vi "Find Connected Resources.vi"(8 "error in (no error)":errorcluster, 9 "Return Aliases":bool=TRUE, 10 "Search Expression":string="?*", 11 "AbstractResourceEnumerator in":refnum<class "AbstractResourceEnumerator.lvclass">) -> (0 "error out":errorcluster, 2 "Found Resources":string[](array[string]), 3 "AbstractResourceEnumerator out":refnum<class "AbstractResourceEnumerator.lvclass">)   [LabVIEW 2023, in "HAF.lvlib" / "AbstractResourceEnumerator.lvclass"]
doc: "Builds a collection of names of resources currently connected to the System. If Return Aliases is True, then only resources with an Alias are returned - any connected resource without an alias is ignored. If Return Aliases is False then the collection will be for all connected resources."
uses:
  AbstractResourceEnumerator.lvclass
  AbstractResourceEnumerator.lvclass/AbstractResourceEnumerator.ctl
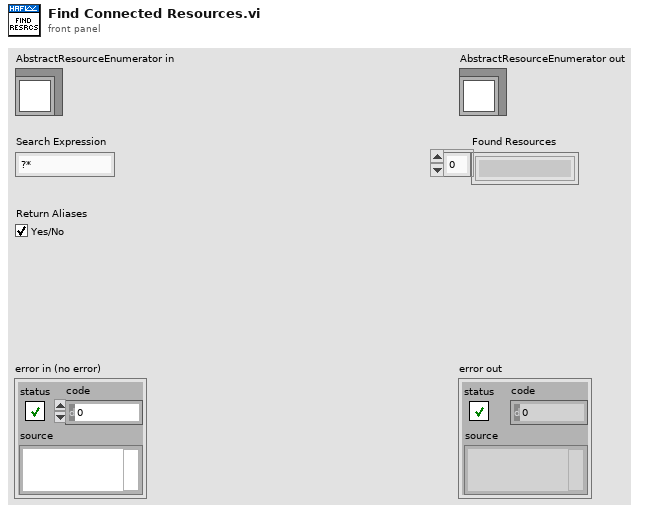
[diagram p1: front panel]
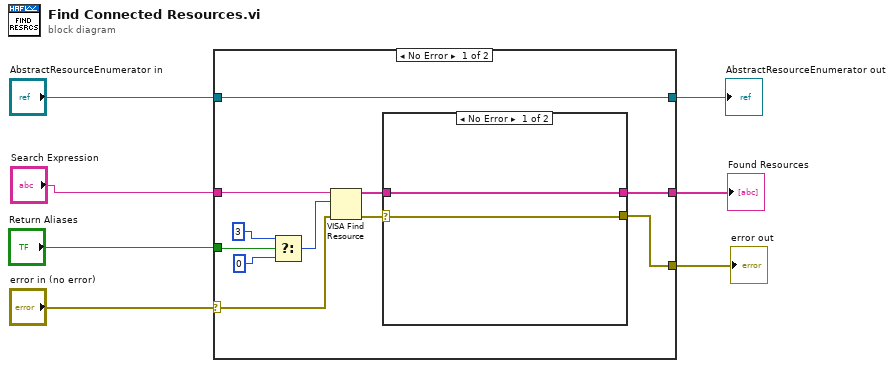
[diagram p0: block diagram]
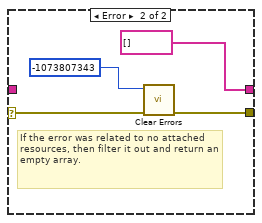
[diagram p2: hidden frame]
diagram:
  n1 = case shown="No Error" "error in (no error)" {
    selector: "error in (no error)" -> [w13 w25]
    tunnel: [w11 w26] -> w3
    tunnel: "AbstractResourceEnumerator in" -> [w11 w26]
    tunnel: "Return Aliases" -> [w18 _]
    tunnel: "Search Expression" -> [w15 _]
    tunnel: [w10 _] -> w2
    tunnel: [w9 w25] -> w1
    frame No Error {
      n2 = Select(t=u32 3, s=w18, f=u32 0) -> (s? t:f=w14:u32)
      n3 = VISA Find Resource(8:w13, 10:w14, 11:w15) -> (0:w8:errorcluster, 3:w12:string[])  [unwired: 1 out]
      n4 = case shown="No Error" w8 {
        selector: w8 -> [w19 w23]
        tunnel: [w19 w22] -> w9
        tunnel: [w20 string[] []] -> w10
        tunnel: w12 -> [w20 _]
        frame No Error {
        }
        frame Error {
          # "If the error was related to no attached resources, then filter it out and return an empty array."
          n5 = call <vilib>:"Clear Errors.vi"("error in (no error)"=w23, "specific error code to clear (0: all)"=-1073807343) -> ("error out"=w22:errorcluster)  [unwired: 4 in, 1 out]
        }
      }
    }
    frame Error {
    }
  }
  "error out" <- w1
  "AbstractResourceEnumerator out" <- w3
  "Found Resources" <- w2
